vi "Set RIO INI Key.vi"(8 "error in (no error)":errorcluster) -> (0 "error out":errorcluster)   [LabVIEW 2015, in "FPGA Addon Engine.lvlib"]
uses:
  FPGA Addon Engine.lvlib
  <vilib>/Utility/config.llb/Write Key (I32).vi
  <vilib>/Utility/config.llb/NI_LVConfig.lvlib
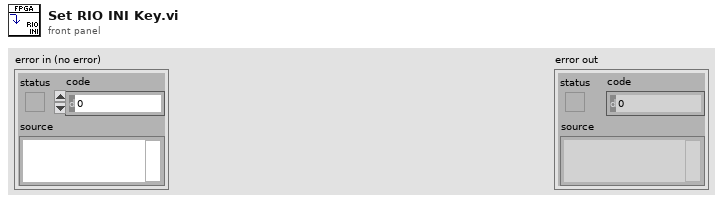
[diagram p1: front panel]
types:
  T1 = typedef "NI_LVConfig.lvlib/Config Data RefNum.ctl" = refnum<k1>
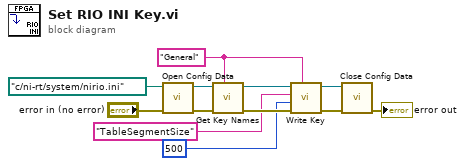
[diagram p0: block diagram]
diagram:
  w9 = "General" ("section")
  n1 = call <vilib>:"Open Config Data.vi"("error in (no error)"="error in (no error)", "configuration file path"=path "c:/ni-rt/system/nirio.ini") -> ("error out"=w12:errorcluster, "refnum"=w11:T1)  [unwired: 7 in, 1 out]
  n2 = call <vilib>:"Get Key Names.vi"("section"=w9, "error in (no error)"=w12, "refnum"=w11) -> ("error out"=w8:errorcluster, "refnum out"=w10:T1)  [unwired: 5 in, 2 out]
  n3 = call-poly <vilib>:"Write Key.vi"("section"=w9, "error in (no error)"=w8, "value"=500, "key"="TableSegmentSize", "refnum"=w10) -> ("error out"=w4:errorcluster, "refnum out"=w7:T1)  [unwired: 4 in, 1 out]
  n4 = call <vilib>:"Close Config Data.vi"("error in (no error)"=w4, "refnum"=w7) -> ("error out"=→"error out":errorcluster)  [unwired: 8 in, 1 out]
